vi "AS_REMOVE.vi"(8 "error in (no error)":errorcluster, 9 "拍攝B讀取條碼":string, 10 "拍攝A讀取條碼":string, 11 "DBLink":string) -> (0 "error out":errorcluster, 2 "下料工件":cluster{"條碼A":string, "條碼B":string}, 3 "Workspace: Assemble":cluster{"條碼A":string, "條碼B":string}[](array[cluster]))   [LabVIEW 2019]
panel:
  out "組合區異常需人員排除":bool
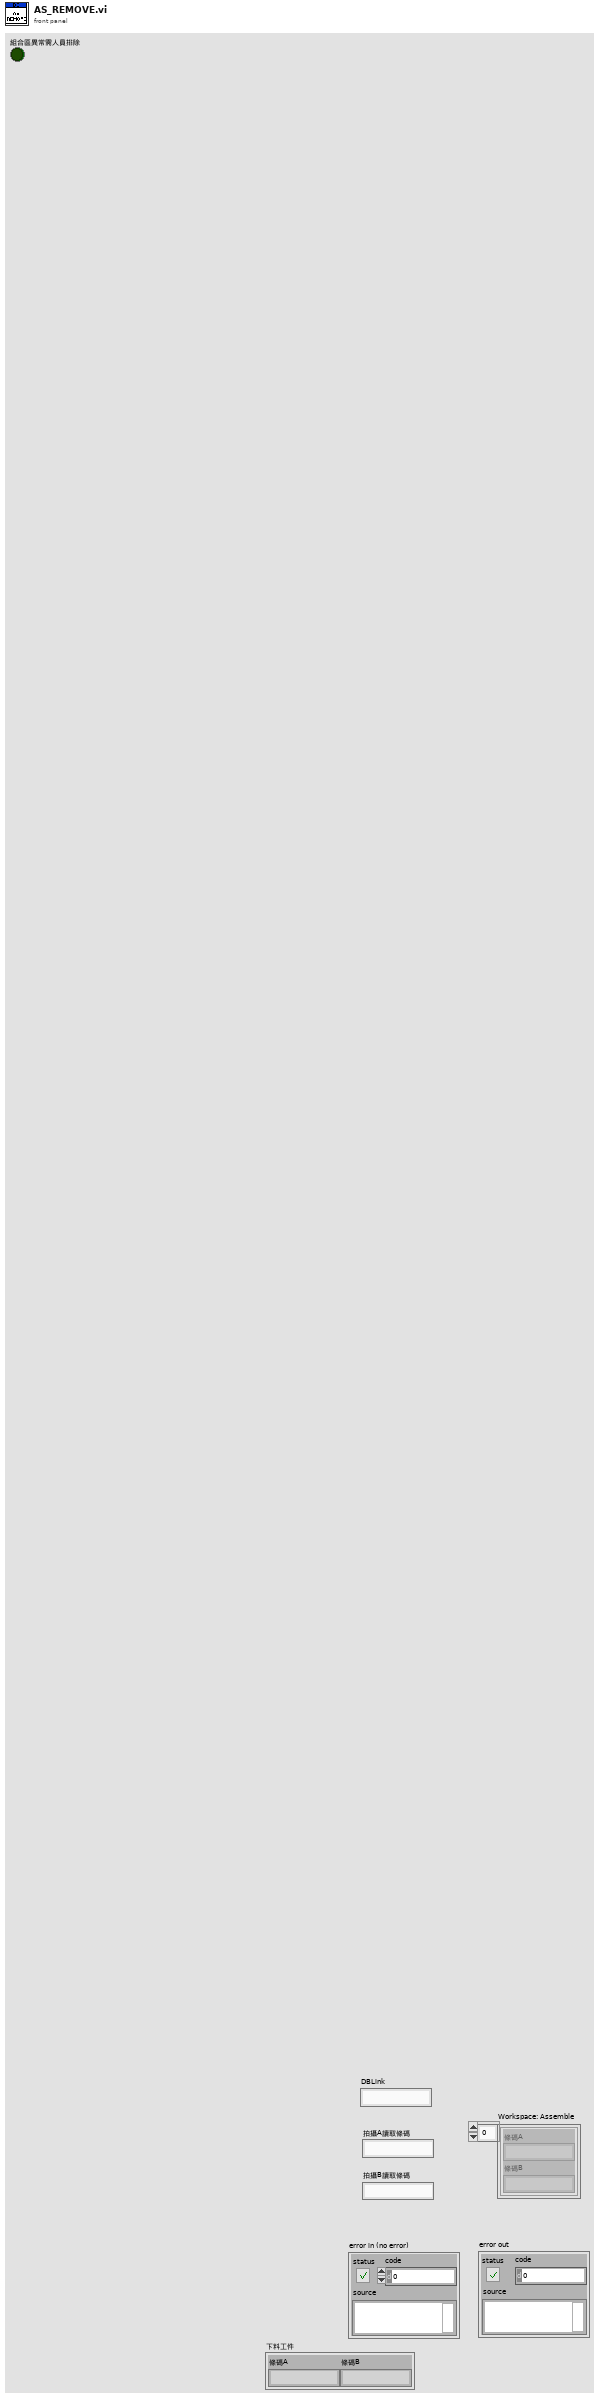
[diagram p1: front panel]
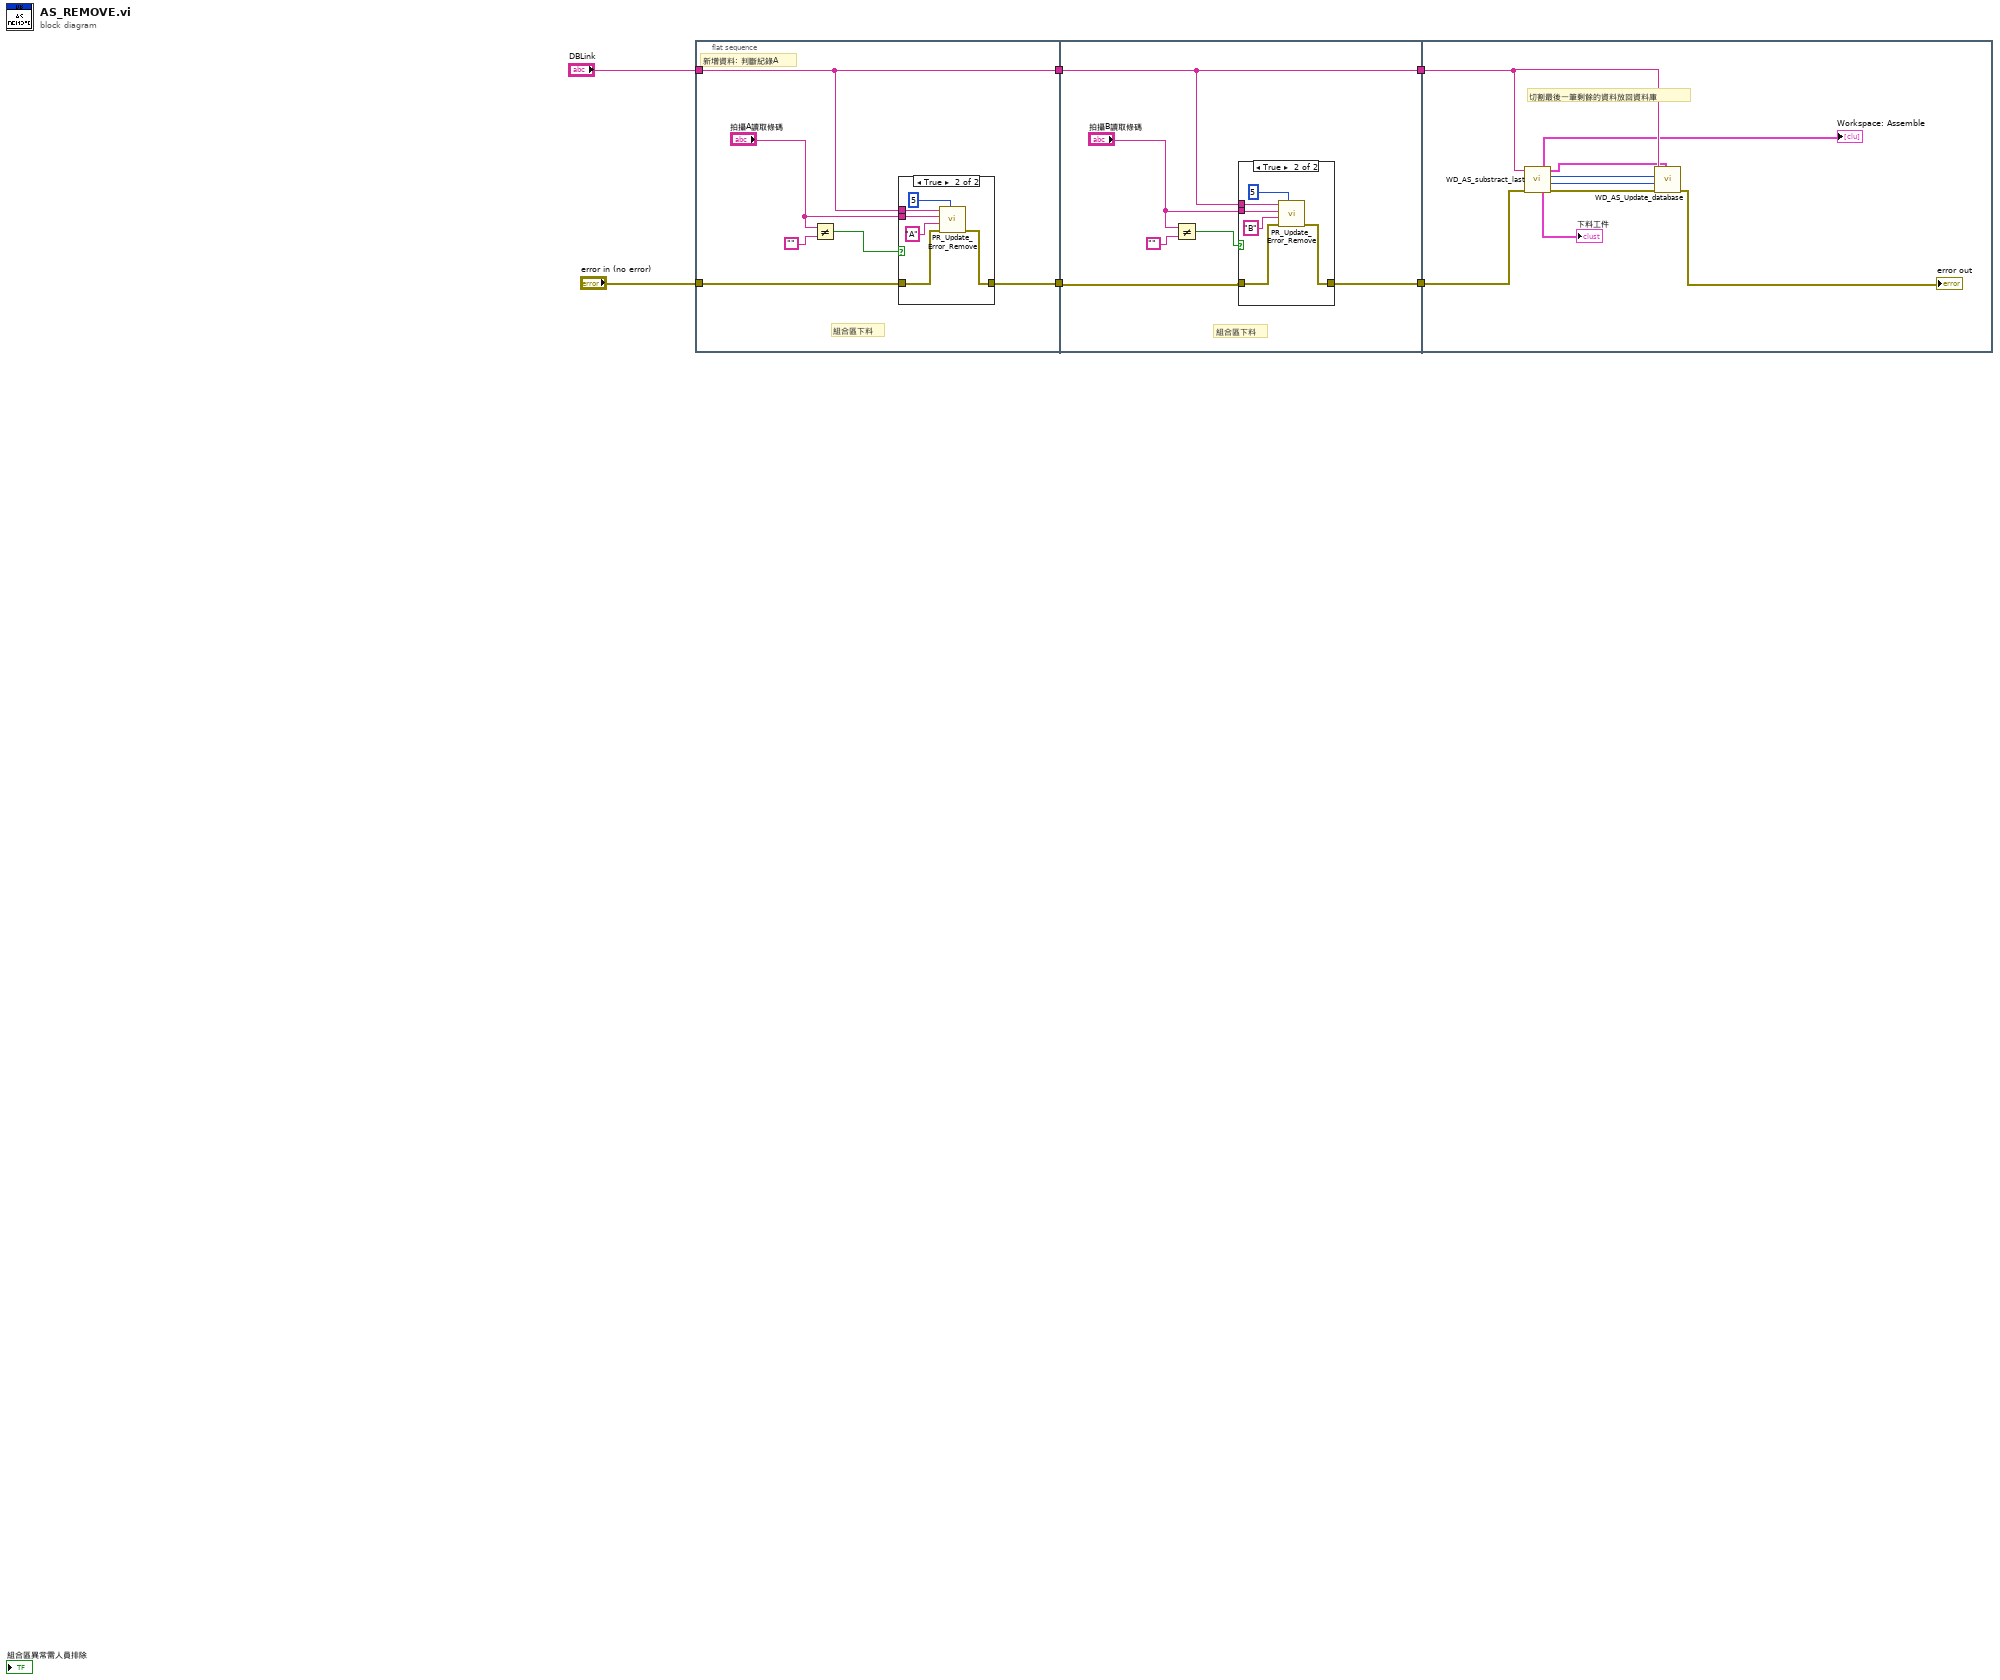
[diagram p0: block diagram]
diagram:
  n1 = flat-sequence {
    tunnel: "DBLink" -> [w11]
    tunnel: [w11] -> w4
    tunnel: "error in (no error)" -> [w9]
    tunnel: [w8] -> w3
    tunnel: w4 -> [w24]
    tunnel: w3 -> [w22]
    tunnel: [w21] -> w2
    tunnel: [w24] -> w1
    tunnel: w2 -> [w40]
    tunnel: w1 -> [w41]
    frame #0 {
      # "組合區下料"
      # "新增資料: 判斷紀錄A"
      n2 = Not Equal?(x="拍攝A讀取條碼", y="") -> (x != y?=w7:bool)
      n3 = case shown="True" w7 {
        tunnel: w11 -> [_ w18]
        tunnel: w9 -> [w13 w16]
        tunnel: [w13 w15] -> w8
        tunnel: "拍攝A讀取條碼" -> [_ w14]
        frame False {
        }
        frame True {
          n4 = call "PR_Update_Error_Remove.vi"("[workplace_id]"=i16 5 ("workspace"), "error in (no error)"=w16, "position"="A" ("pos"), "barcode"=w14, "DBlink"=w18) -> ("error out"=w15:errorcluster)  [unwired: 6 in]
        }
      }
    }
    frame #1 {
      # "組合區下料"
      n5 = Not Equal?(x="拍攝B讀取條碼", y="") -> (x != y?=w20:bool)
      n6 = case shown="True" w20 {
        tunnel: w24 -> [_ w31]
        tunnel: w22 -> [w26 w29]
        tunnel: [w26 w28] -> w21
        tunnel: "拍攝B讀取條碼" -> [_ w27]
        frame False {
        }
        frame True {
          n7 = call "PR_Update_Error_Remove.vi"("[workplace_id]"=i16 5 ("workspace"), "error in (no error)"=w29, "position"="B" ("pos"), "barcode"=w27, "DBlink"=w31) -> ("error out"=w28:errorcluster)  [unwired: 6 in]
        }
      }
    }
    frame #2 {
      # "切割最後一筆剩餘的資料放回資料庫"
      n8 = call "WD_AS_substract_last.vi"("error in (no error)"=w40, "DBLink"=w41) -> ("error out"=w35:errorcluster, "站點總數"=w36:i32, "當前料數"=w37:i32, "計算用 array"=w38:cluster{"條碼A":string, "條碼B":string}[], "取出element"=→"下料工件":cluster{"條碼A":string, "條碼B":string}, "顯示用array"=→"Workspace: Assemble":cluster{"條碼A":string, "條碼B":string}[])  [unwired: 4 in]
      n9 = call "WD_AS_Update_database.vi"("計算用array"=w38, "error in (no error)"=w35, "站點總數"=w36, "當前料數"=w37, "DBLink"=w41) -> ("error out"=→"error out":errorcluster)  [unwired: 6 in]
    }
  }
